vi "Write String.vi"(8 "error in (no error)":errorcluster, 10 "String":string, 11 "Refnum in":T1) -> (0 "error out":errorcluster, 3 "Refnum out":T1)   [LabVIEW 2019, in "HD44780.lvlib"]
uses:
  HD44780.lvlib
  FPGA VI Reference.ctl
  <vilib>/Utility/error.llb/Error Cluster From Error Code.vi
  <vilib>/rvi/errors/niLvFpgaAdjustHostInterfaceError.vi
  <vilib>/rvi/interface/nirviReadWriteControl/nirviReadWriteControl.xnode
  NiFpgaLv.dll
  <vilib>/rvi/interface/Simulation/niFpgaSimulationCallBeginRW.vi
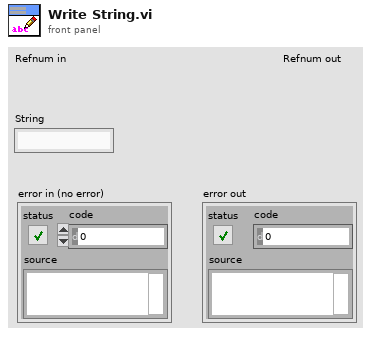
[diagram p1: front panel]
types:
  T1 = typedef "FPGA VI Reference.ctl" = refnum<k20>
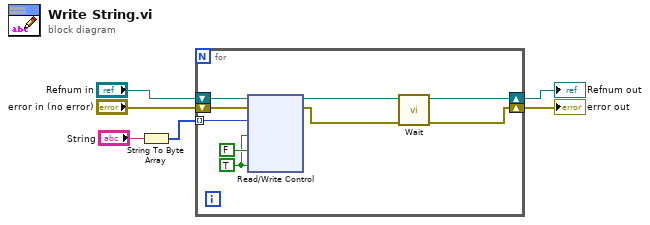
[diagram p0: block diagram]
diagram:
  n1 = String To Byte Array(string="String") -> (unsigned byte array=w1:u8[])
  n2 = for {
    tunnel: w1 -> [w11] mode=indexing
    shift-right: [w8] -> w6
    shift-left: "error in (no error)" -> [w14]
    shift-right: [w7] -> w5
    shift-left: "Refnum in" -> [w13]
    w12 = TRUE ("Enable")
    n3 = xnode "Read/Write Control"("FPGA VI Reference In"=w13, "error in"=w14, "Data In"=w11, "RS"=w12, "R/W"=FALSE ("RS"), "Enable"=w12) -> ("FPGA VI Reference Out"=w10:T1, "error out"=w9:errorcluster)
    n4 = call "Wait.vi"("error in (no error)"=w9, "Refnum in"=w10) -> ("error out"=w8:errorcluster, "Refnum out"=w7:T1)  [unwired: 8 in]
  }
  "error out" <- w6
  "Refnum out" <- w5
